vi "Calculate parameters API.vi"(7 "Scope":T1={"Config"={"VISA Resource"="", "Model"=enum."DPO 3012", "Timebase"=0.0, "Timeout (ms)"=0, "TAS"={"Vertical Range (V)"=0.0, "Vertical Offset (0.0 divs)"=0.0, "Bandwidth"=0, "Probe Attenuation (10.0)"=0.0, "Vertical Coupling"=0, "Impedance"=0, "Multiplication factor"=0.0, "Channel"=enum."Channel 1"}, "TPC"={"Vertical Range (V)"=0.0, "Vertical Offset (0.0 divs)"=0.0, "Bandwidth"=0, "Probe Attenuation (10.0)"=0.0, "Vertical Coupling"=0, "Impedance"=0, "Multiplication factor"=0.0, "Channel"=enum."Channel 1"}, "Trigger"={"Mode"=enum."Laser (TAS)", "Source "=enum."Channel 1", "PIA"={"Test LEDs"=FALSE, "LED line"="", "LED off (s)"=0.0, "LED on (s)"=0.0}, "Threshold (V)"=0.0004}}, "Indicators"={"Setup"={"Final number of points"=0.0, "Pretrigger points"=0.0, "Number of readouts"=0, "Model"={"Acquisition Type"=0, "Record length (points)"=0, "Averages on scope"=0, "Average number of points"=0.0}}, "Timestamp of Data"=timestamp(0 s since 1904-01-01)}, "Data"={"TPC"={"Live data"={"t0"=timestamp(0 s since 1904-01-01), "dt"=1.0, "Y"=[]}, "Averaged data"={"t0"=timestamp(0 s since 1904-01-01), "dt"=1.0, "Y"=[]}, "Accumulated data"={"t0"=timestamp(0 s since 1904-01-01), "dt"=1.0, "Y"=[]}, "Final data"={"t0"=timestamp(0 s since 1904-01-01), "dt"=1.0, "Y"=[]}}, "TAS"={"Live data"={"t0"=timestamp(0 s since 1904-01-01), "dt"=1.0, "Y"=[]}, "Averaged data"={"t0"=timestamp(0 s since 1904-01-01), "dt"=1.0, "Y"=[]}, "Accumulated data"={"t0"=timestamp(0 s since 1904-01-01), "dt"=1.0, "Y"=[]}, "Final data"={"t0"=timestamp(0 s since 1904-01-01), "dt"=1.0, "Y"=[]}}, "Time arrays"={"Time array (decimated)"=[], "waveform"={"t0"=timestamp(0 s since 1904-01-01), "dt"=1.0, "Y"=[]}}}, "Test"={"Config"={"Amplification Factor"=2.0, "100% Reflectance Standard"=2.0, "Calculation Method"=enum."Reflectance", "Option to discard new data?"=FALSE, "Mode"=enum."Spectrum", "Number of Averages"=0, "B Test?"=FALSE}, "Indicators"={"DAQ Background Level (V)"=2.0, "A-Test Counter"=2, "B-Test Counter"=2, "Type"=enum."A-Test", "Scope Background Level (Amps)"=2.0, "TAS only?"=FALSE}}} {"Test"."Config"."Number of Averages" min=0; "Indicators"."Setup"."Model"."Record length (points)" items=["1000"=1, "10,000"=10, "100,000"=100, "1,000,000"=1000, "5,000,000"=5000, "10,000,000"=10000]; "Indicators"."Setup"."Model"."Acquisition Type" items=["Sample", "Peak Detect", "Hi Res", "Envelope", "Average"]; "Config"."Trigger"."Threshold (V)" format="%#_3f"; "Config"."TPC"."Impedance" items=["1M", "75", "50"]; "Config"."TPC"."Vertical Coupling" items=["AC", "DC", "Ground"]; "Config"."TPC"."Bandwidth" items=["FULL", "250 MHz", "150 MHz", "20 MHz"]; "Config"."TAS"."Impedance" items=["1M", "75", "50"]; "Config"."TAS"."Vertical Coupling" items=["AC", "DC", "Ground"]; "Config"."TAS"."Bandwidth" items=["FULL", "250 MHz", "150 MHz", "20 MHz"]; "Config"."Timebase" format="%^#_3e"}, 8 "Error In":errorcluster) -> (0 "Error Out":errorcluster)   [LabVIEW 2017, in "Scope.lvlib"]
uses:
  Scope.lvlib
  Controls/Params.ctl
  Controls/Models.ctl
  Controls/TPC.ctl
  Controls/Channels.ctl
  Trigger/Controls/Params.ctl
  Trigger/Controls/Mode.ctl
  Trigger/Controls/Trigger channels.ctl
  Controls/Acquisition type.ctl
  Controls/Record length.ctl
  Controls/Data.ctl
  Controls/Channel data.ctl
  System Control/CTLs/Test params.ctl
  System Control/CTLs/Test Controls.ctl
  System Control/CTLs/Test indicators.ctl
  System Control/CTLs/Test Type.ctl
  Controls/Command Data [cluster].ctl
  Controls/Commands [enum].ctl
  Events/Events.lvlib
  Trigger/Trigger.lvlib
  System Control/Main controller.lvlib
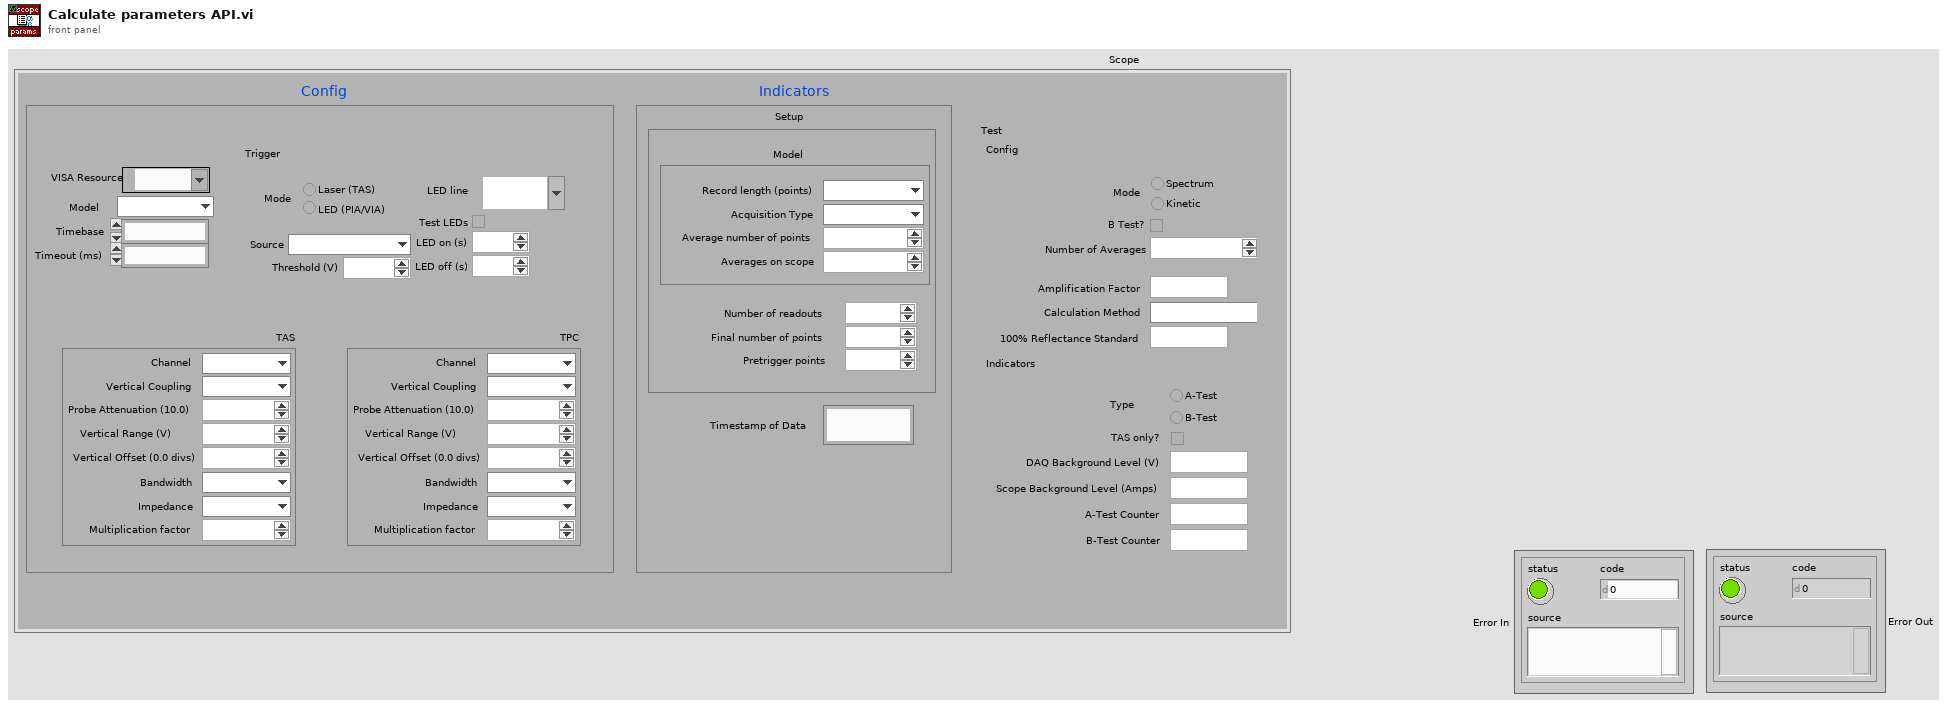
[diagram p1: front panel]
types:
  T1 = typedef "Scope.lvlib/Params.ctl" = cluster{"Config":cluster{"VISA Resource":refnum<visa-resource-name>, "Model":T2, "Timebase":dbl, "Timeout (ms)":u32, "TAS":T3, "TPC":T3, "Trigger":T5}, "Indicators":cluster{"Setup":cluster{"Final number of points":dbl, "Pretrigger points":dbl, "Number of readouts":i32, "Model":cluster{"Acquisition Type":T8, "Record length (points)":T9, "Averages on scope":i32, "Average number of points":dbl}}, "Timestamp of Data":timestamp}, "Data":T10, "Test":T12}
  T2 = typedef "Scope.lvlib/Models.ctl" = enum16{"DPO 3012", "DPO 2012B", "TDS 3012C"}
  T3 = typedef "Scope.lvlib/TPC.ctl" = cluster{"Vertical Range (V)":dbl, "Vertical Offset (0.0 divs)":dbl, "Bandwidth":i32, "Probe Attenuation (10.0)":dbl, "Vertical Coupling":u16, "Impedance":u16, "Multiplication factor":dbl, "Channel":T4}
  T4 = typedef "Scope.lvlib/Channels.ctl" = enum16{"Channel 1", "Channel 2", "Channel 3", "Channel 4", "Math", "Reference A", "Reference B", "Reference C", "Reference D", "B1", "B2", "None"}
  T5 = typedef "Scope.lvlib/Trigger.lvlib/Params.ctl" = cluster{"Mode":T6, "Source ":T7, "PIA":cluster{"Test LEDs":bool, "LED line":tag, "LED off (s)":dbl, "LED on (s)":dbl}, "Threshold (V)":dbl}
  T6 = typedef "Scope.lvlib/Trigger.lvlib/Mode.ctl" = enum32{"Laser (TAS)", "LED (PIA/VIA)"}
  T7 = typedef "Scope.lvlib/Trigger.lvlib/Trigger channels.ctl" = enum16{"Channel 1", "Channel 2", "Channel 3", "Channel 4", "AC Line", "Aux", "Digital Channel 0", "Digital Channel 1", "Digital Channel 2", "Digital Channel 3", "Digital Channel 4", "Digital Channel 5", "Digital Channel 6", "Digital Channel 7", "Digital Channel 8", "Digital Channel 9", "Digital Channel 10", "Digital Channel 11", "Digital Channel 12", "Digital Channel 13", "Digital Channel 14", "Digital Channel 15", "RF"}
  T8 = typedef "Scope.lvlib/Acquisition type.ctl" = u16
  T9 = typedef "Scope.lvlib/Record length.ctl" = u32
  T10 = typedef "Scope.lvlib/Data.ctl" = cluster{"TPC":T11, "TAS":T11, "Time arrays":cluster{"Time array (decimated)":dbl[], "waveform":waveform(dbl)}}
  T11 = typedef "Scope.lvlib/Channel data.ctl" = cluster{"Live data":waveform(dbl), "Averaged data":waveform(dbl), "Accumulated data":waveform(dbl), "Final data":waveform(dbl)}
  T12 = typedef "Main controller.lvlib/Test params.ctl" = cluster{"Config":T13, "Indicators":T14}
  T13 = typedef "Main controller.lvlib/Test Controls.ctl" = cluster{"Amplification Factor":dbl, "100% Reflectance Standard":dbl, "Calculation Method":enum16{"Reflectance", "Transmission", "Kubelka-Munk"}, "Option to discard new data?":bool, "Mode":enum32{"Spectrum", "Kinetic"}, "Number of Averages":i32, "B Test?":bool}
  T14 = typedef "Main controller.lvlib/Test indicators.ctl" = cluster{"DAQ Background Level (V)":dbl, "A-Test Counter":i32, "B-Test Counter":i32, "Type":T15, "Scope Background Level (Amps)":dbl, "TAS only?":bool}
  T15 = typedef "Main controller.lvlib/Test Type.ctl" = enum32{"A-Test", "B-Test"}
  T16 = typedef "Scope.lvlib/Command Data [cluster].ctl" = cluster{"Command":T17, "Data":variant}
  T17 = typedef "Scope.lvlib/Commands [enum].ctl" = enum16{"Calculate parameters", "Start", "Stop", "Send data", "Start acquisition", "Get test data", "Accumulate test data", "Average test data", "Add background voltage", "Scale TPC", "Average Pre Trigger Data", "Write to file"}
  T18 = typedef "Events.lvlib/Refs [cluster].ctl" = cluster{"Exit":refnum<user-event>, "Controller":refnum<user-event>, "System Error":refnum<user-event>, "UI":refnum<user-event>, "Example Module":refnum<user-event>, "Shutter":refnum<user-event>, "Monochromator":refnum<user-event>, "DAQ":refnum<user-event>, "Scope":refnum<user-event>, "Processing":refnum<user-event>, "File IO":refnum<user-event>, "Colour wheel":refnum<user-event>}
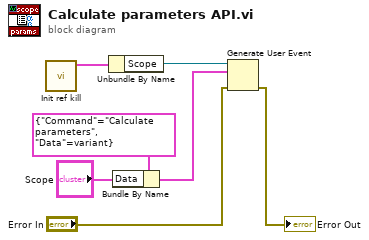
[diagram p0: block diagram]
diagram:
  n1 = call "Init ref kill.vi"() -> ("Messages"=w7:T18)  [unwired: 10 in, 1 out]
  n2 = Unbundle By Name(w7) -> ("Scope"=w6:refnum<user-event>)
  n3 = Bundle By Name(cluster=T16 {"Command"=enum."Calculate parameters", "Data"=variant} ("event data"), "Data"="Scope") -> (w3:T16)
  n4 = Generate User Event(user event=w6, event data cluster=w3, error in="Error In") -> (error out=→"Error Out":errorcluster)  [unwired: 1 in, 1 out]
